vi "Reshape Byte Array.vi"(8 "error in (no error)":errorcluster, 10 "FrameDescription":T1, 11 "Byte Array":u8[](array[numeric])) -> (0 "error out":errorcluster, 3 "2D Array":u8[][](array[numeric]))   [LabVIEW 2011, in "LVH-KinectOne.lvlib"]
uses:
  LVH-KinectOne.lvlib
  Type Defs/FrameDescription.ctl
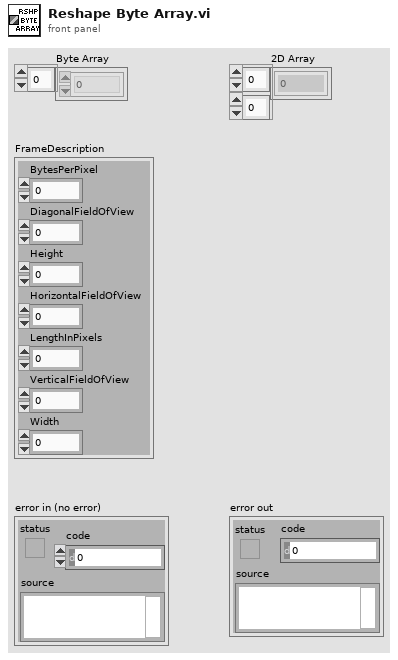
[diagram p1: front panel]
types:
  T1 = typedef "LVH-KinectOne.lvlib/FrameDescription.ctl" = cluster{"BytesPerPixel":u32, "DiagonalFieldOfView":sgl, "Height":i32, "HorizontalFieldOfView":sgl, "LengthInPixels":u32, "VerticalFieldOfView":sgl, "Width":i32}
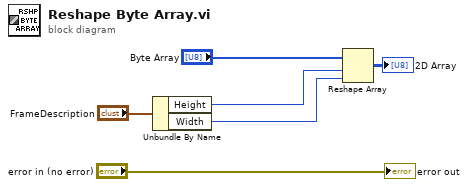
[diagram p0: block diagram]
diagram:
  n1 = Unbundle By Name("FrameDescription") -> ("Height"=w5:i32, "Width"=w4:i32)
  n2 = Reshape Array("Byte Array", w5, w4) -> (→"2D Array":u8[][])
  "error out" <- "error in (no error)"
